vi "VI Tree.vi"   [LabVIEW 2009, in "Zurich Instruments LabOne.lvlib"]
doc: "This is the instrument driver for the <INSTRUMENT NAME>. The VI Tree displays all the user-callable VIs of the instrument driver in an organized table."
uses:
  <instrlib>/Zurich Instruments LabOne/Zurich Instruments LabOne.lvlib
  <instrlib>/Zurich Instruments LabOne/Public/Configure/ziGetValueDouble.vi
  <instrlib>/Zurich Instruments LabOne/Public/Configure/ziSetValueDouble.vi
  <instrlib>/Zurich Instruments LabOne/Public/Modules/ziModSetValueBinary.vi
  <instrlib>/Zurich Instruments LabOne/Public/Modules/ziModGetDoubleData.vi
  <instrlib>/Zurich Instruments LabOne/Public/Utility/ziTicksToS_single.vi
  <instrlib>/Zurich Instruments LabOne/Public/Data/ziGetEventAuxInSample.vi
  <instrlib>/Zurich Instruments LabOne/Public/Modules/ziModGetNodeValueDouble.vi
panel:
  # "(c) 2009-2014 Zurich Instruments.  ALL RIGHTS RESERVED."
  # "SEE DIAGRAM\nFOR VI TREE."
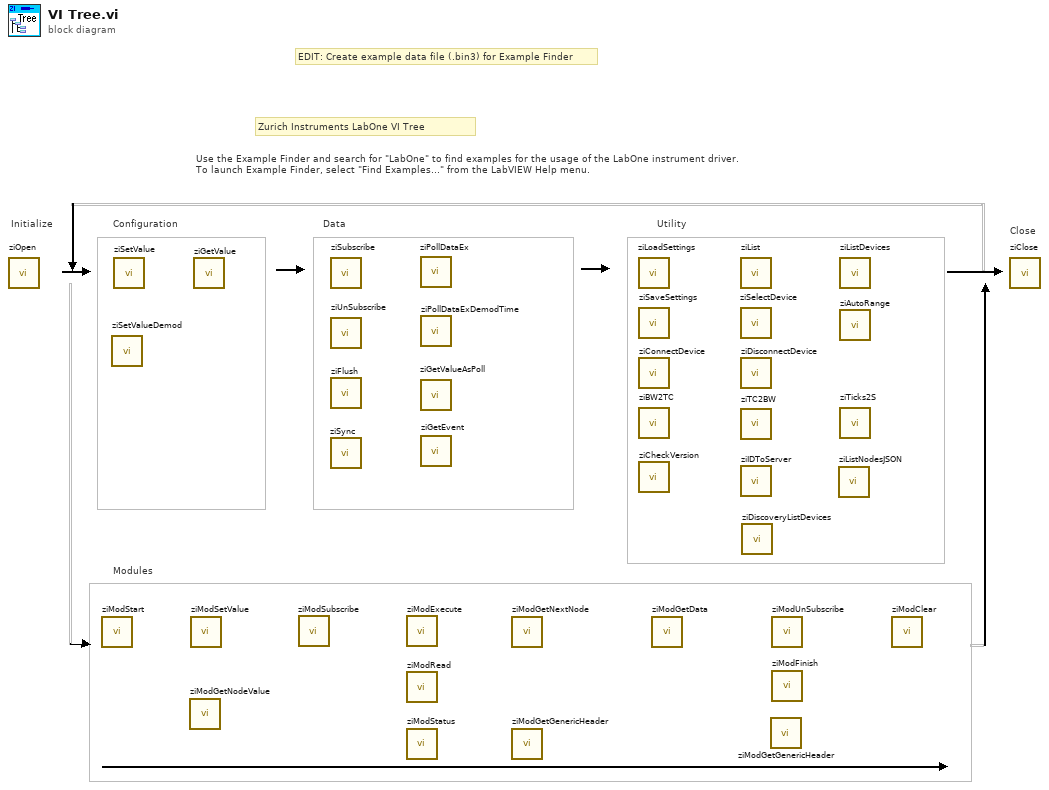
[diagram p0: block diagram]
diagram:
  # "Modules"
  # "Zurich Instruments LabOne VI Tree"
  # "EDIT: Create example data file (.bin3) for Example Finder"
  # "Use the Example Finder and search for \"LabOne\" to find examples for the usage of the LabOne instrument driver.\nTo launch Example Finder, select \"Find Examples...\" from the LabVIEW Help menu."
  # "Configuration"
  # "Utility"
  # "Data"
  # "Close"
  # "Initialize"
  n1 = call <instrlib>:"ziOpen.vi"() -> ()  [unwired: 4 in, 3 out]
  n2 = call <instrlib>:"ziModStart.vi"() -> ()  [unwired: 9 in, 3 out]
  n3 = call <instrlib>:"ziSetValueDemod.vi"() -> ()  [unwired: 10 in, 2 out]
  n4 = call-poly <instrlib>:"ziSetValue.vi"() -> ()  [unwired: 5 in, 2 out]
  n5 = call-poly <instrlib>:"ziModGetNodeValue.vi"() -> ()  [unwired: 13 in, 3 out]
  n6 = call-poly <instrlib>:"ziModSetValue.vi"() -> ()  [unwired: 10 in, 2 out]
  n7 = call-poly <instrlib>:"ziGetValue.vi"() -> ()  [unwired: 3 in, 3 out]
  n8 = call <instrlib>:"ziModSubscribe.vi"() -> ()  [unwired: 9 in, 2 out]
  n9 = call <instrlib>:"ziSubscribe.vi"() -> ()  [unwired: 4 in, 2 out]
  n10 = call <instrlib>:"ziUnSubscribe.vi"() -> ()  [unwired: 4 in, 2 out]
  n11 = call <instrlib>:"ziFlush.vi"() -> ()  [unwired: 10 in, 2 out]
  n12 = call <instrlib>:"ziSync.vi"() -> ()  [unwired: 14 in, 2 out]
  n13 = call <instrlib>:"ziModExecute.vi"() -> ()  [unwired: 8 in, 3 out]
  n14 = call <instrlib>:"ziModRead.vi"() -> ()  [unwired: 10 in, 2 out]
  n15 = call <instrlib>:"ziModStatus.vi"() -> ()  [unwired: 7 in, 4 out]
  n16 = call <instrlib>:"ziPollDataEx.vi"() -> ()  [unwired: 4 in, 8 out]
  n17 = call <instrlib>:"ziPollDataExDemodTime.vi"() -> ()  [unwired: 9 in, 3 out]
  n18 = call <instrlib>:"ziGetValueAsPoll.vi"() -> ()  [unwired: 4 in, 2 out]
  n19 = call-poly <instrlib>:"ziGetEvent.vi"() -> ()  [unwired: 9 in, 3 out]
  n20 = call <instrlib>:"ziModGetNextNode.vi"() -> ()  [unwired: 8 in, 4 out]
  n21 = call <instrlib>:"ziModGetGenericHeader.vi"() -> ()  [unwired: 9 in, 3 out]
  n22 = call <instrlib>:"ziLoadSettings.vi"() -> ()  [unwired: 5 in, 2 out]
  n23 = call <instrlib>:"ziSaveSettings.vi"() -> ()  [unwired: 4 in, 3 out]
  n24 = call <instrlib>:"ziConnectDevice.vi"() -> ()  [unwired: 10 in, 2 out]
  n25 = call <instrlib>:"ziBW2TC.vi"() -> ()  [unwired: 3 in, 1 out]
  n26 = call <instrlib>:"ziCheckVersion.vi"() -> ()  [unwired: 13 in, 3 out]
  n27 = call-poly <instrlib>:"ziModGetData.vi"() -> ()  [unwired: 7 in, 5 out]
  n28 = call <instrlib>:"ziList.vi"() -> ()  [unwired: 4 in, 3 out]
  n29 = call <instrlib>:"ziSelectDevice.vi"() -> ()  [unwired: 3 in, 3 out]
  n30 = call <instrlib>:"ziDisconnectDevice.vi"() -> ()  [unwired: 10 in, 2 out]
  n31 = call <instrlib>:"ziTC2BW.vi"() -> ()  [unwired: 3 in, 1 out]
  n32 = call <instrlib>:"ziIDToServer.vi"() -> ()  [unwired: 13 in, 3 out]
  n33 = call <instrlib>:"ziDiscoveryListDevices.vi"() -> ()  [unwired: 9 in, 3 out]
  n34 = call <instrlib>:"ziModGetGenericHeader.vi"() -> ()  [unwired: 9 in, 3 out]
  n35 = call <instrlib>:"ziModUnSubscribe.vi"() -> ()  [unwired: 10 in, 2 out]
  n36 = call <instrlib>:"ziModFinish.vi"() -> ()  [unwired: 9 in, 2 out]
  n37 = call <instrlib>:"ziListNodesJSON.vi"() -> ()  [unwired: 13 in, 3 out]
  n38 = call <instrlib>:"ziListDevices.vi"() -> ()  [unwired: 5 in, 3 out]
  n39 = call <instrlib>:"ziAutoRange.vi"() -> ()  [unwired: 9 in, 3 out]
  n40 = call-poly <instrlib>:"ziTicks2S.vi"() -> ()  [unwired: 3 in, 3 out]
  n41 = call <instrlib>:"ziModClear.vi"() -> ()  [unwired: 9 in, 2 out]
  n42 = call <instrlib>:"ziClose.vi"() -> ()  [unwired: 4 in, 2 out]
